vi "ManMarkZagueiro.vi"(8 "Our Robot":T1={"id"=0, "function"=enum."Attacker", "x"=0.0, "y"=0.0, "orientation"=0.0, "v_tangent"=0.0, "v_normal"=0.0, "v_ang"=0.0, "kick_x"=0.0, "kick_z"=0.0, "dribble"=FALSE, "Timestamp"=timestamp(0 s since 1904-01-01), "estimatives"={"est_v_tangent"=0.0, "est_v_normal"=0.0, "est_vx"=0.0, "est_vy"=0.0, "Pos Robot Est"=[]}, "dest_x_kick"=0.0, "dest_y_kick"=0.0, "Gap Coord"=[], "States"=enum."GoToTangent", "Path "=[], "Path  Smooth"=[], "Dest"=[]}, 10 "IA Input":T6={"our_robots"=[], "enemy_robots"=[], "balls"=[], "geometry"={"line_width"=0, "field_length"=0, "field_width"=0, "boundary_width"=0, "referee_width"=0, "goal_width"=0, "goal_depth"=0, "goal_wall_width"=0, "center_circle_radius"=0, "defense_radius"=0, "defense_stretch"=0, "free_kick_from_defense_dist"=0, "penalty_spot_from_field_line_dist"=0, "penalty_line_from_spot_dist"=0}, "IA Judge"={"stage"="", "command"="", "our_goalie_id"=0.0, "enemy_goalie_id"=0.0, "command enum"=enum."Halt", "Time"=enum."Azul"}, "Received Timestamp"=timestamp(0 s since 1904-01-01), "Events"={"Touch"=FALSE, "Ball out"=FALSE, "id touch"=0.0, "Ball out of \nVision"=FALSE, "Ball inside \nGoalie area"=FALSE, "Robot not responding"=FALSE, "Robots responding status"=[1.0, 1.0, 1.0, 1.0, 1.0, 1.0], "Enemy Ball \nPossession"=FALSE, "Pass State"=FALSE, "id end of pass"=0.0, "Kick"=FALSE, "Id ini Possession"=0.0, "Ball Possesion"=FALSE, "Id Possesion"=0.0}}) -> (2 "Robot out":T1={"id"=0, "function"=enum."Attacker", "x"=0.0, "y"=0.0, "orientation"=0.0, "v_tangent"=0.0, "v_normal"=0.0, "v_ang"=0.0, "kick_x"=0.0, "kick_z"=0.0, "dribble"=FALSE, "Timestamp"=timestamp(0 s since 1904-01-01), "estimatives"={"est_v_tangent"=0.0, "est_v_normal"=0.0, "est_vx"=0.0, "est_vy"=0.0, "Pos Robot Est"=[]}, "dest_x_kick"=0.0, "dest_y_kick"=0.0, "Gap Coord"=[], "States"=enum."GoToTangent", "Path "=[], "Path  Smooth"=[], "Dest"=[]})   [LabVIEW 2017]
uses:
  Core/AI Input.ctl
  Core/AI Robot.ctl
  Functions Enum.ctl
  AttackerStates.ctl
  Path Planning/RRT/PathDests.ctl
  Path Planning/RRT/PathDest.ctl
  Core/AI Ball.ctl
  Core/Field Size.ctl
  Core/AI Judge.ctl
  Command Enum.ctl
  Util/Events/Events.ctl
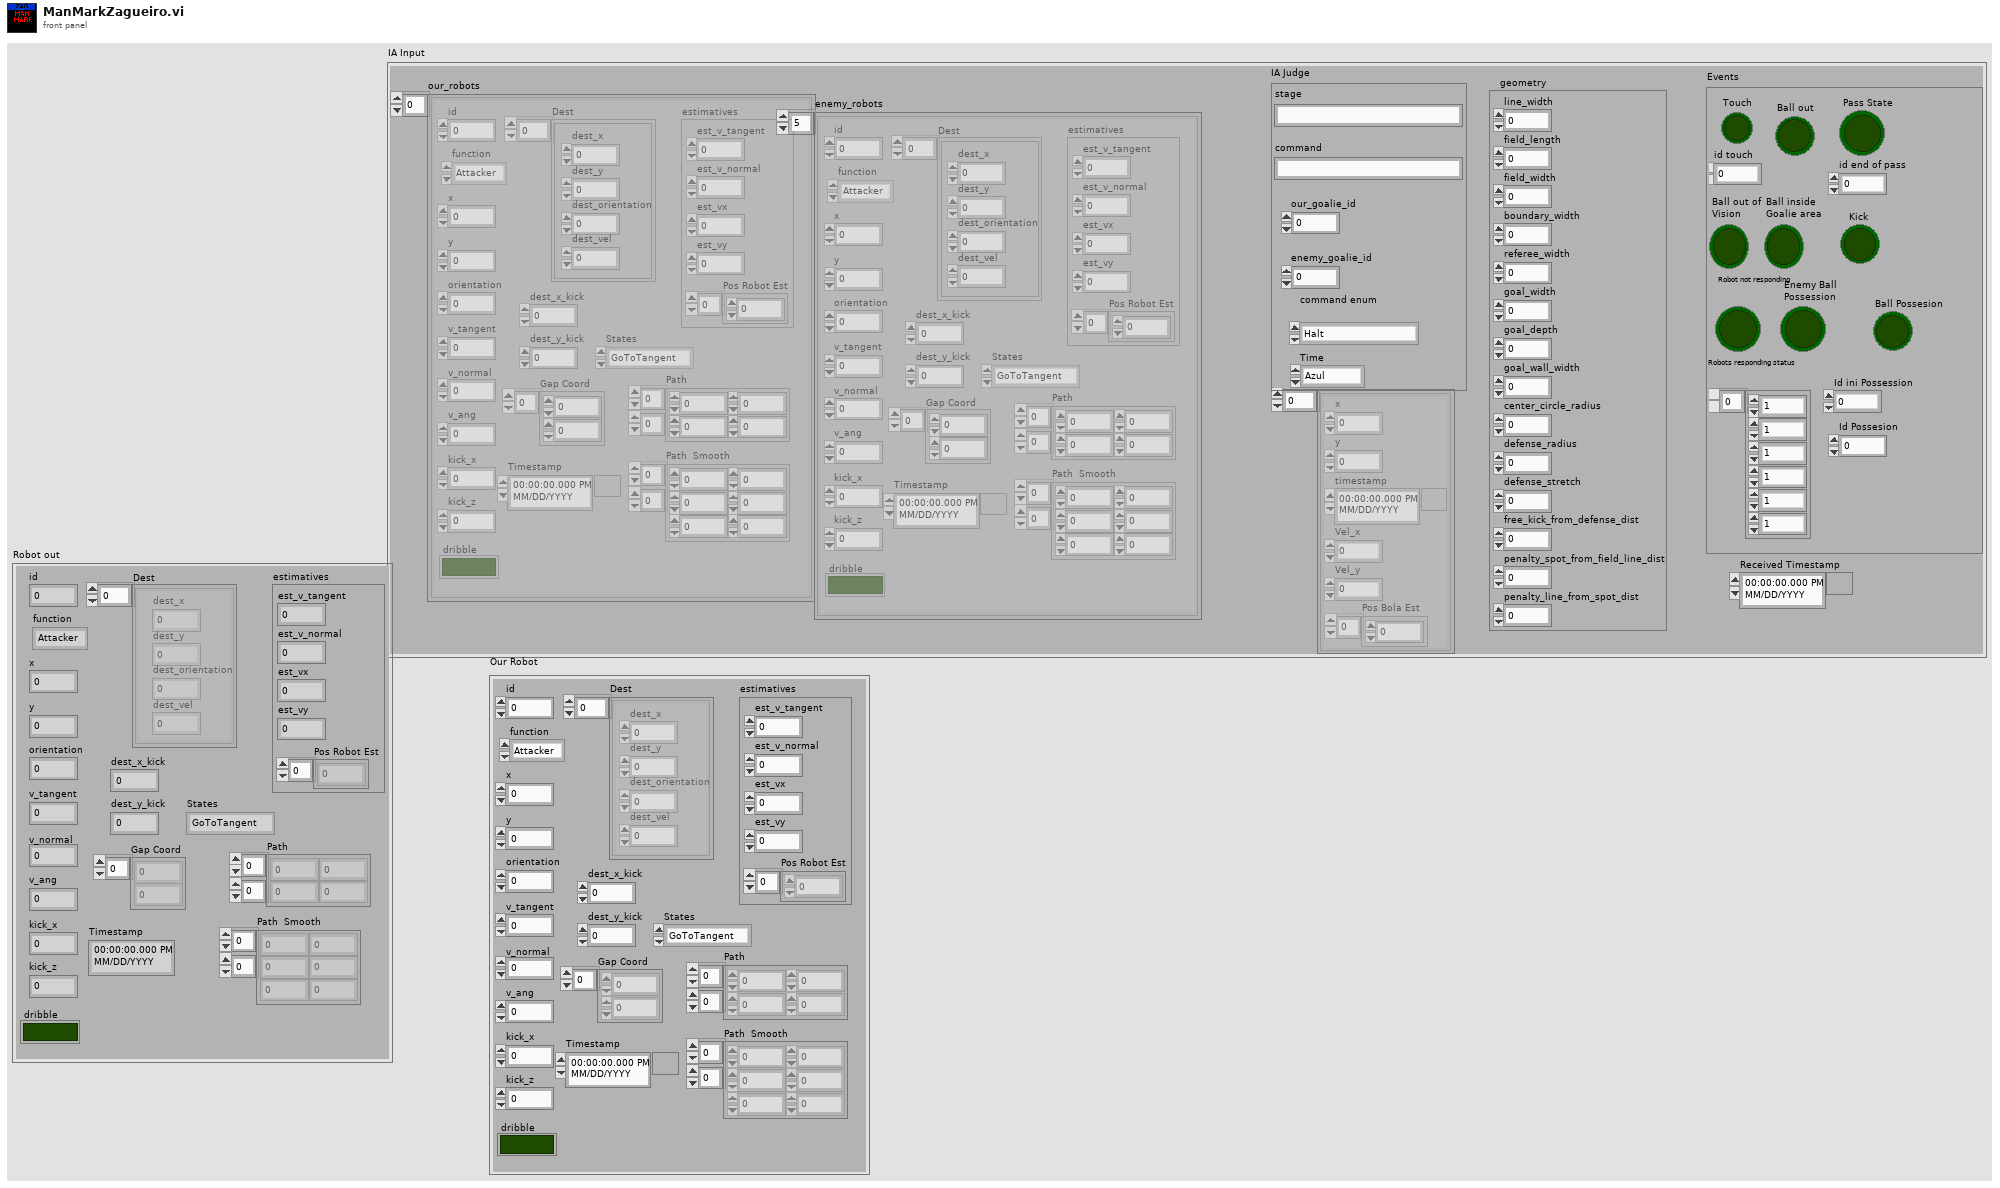
[diagram p1: front panel]
types:
  T1 = typedef "AI Robot.ctl" = cluster{"id":u32, "function":T2, "x":dbl, "y":dbl, "orientation":dbl, "v_tangent":dbl, "v_normal":dbl, "v_ang":dbl, "kick_x":dbl, "kick_z":dbl, "dribble":bool, "Timestamp":timestamp, "estimatives":cluster{"est_v_tangent":dbl, "est_v_normal":dbl, "est_vx":dbl, "est_vy":dbl, "Pos Robot Est":dbl[]}, "dest_x_kick":dbl, "dest_y_kick":dbl, "Gap Coord":dbl[], "States":T3, "Path ":dbl[][], "Path  Smooth":dbl[][], "Dest":T4}
  T2 = typedef "Functions Enum.ctl" = enum16{"Attacker", "Goalie", "Defender", "Striker", "Goto 0", "Dummy", "Kicker", "ZigZag"}
  T3 = typedef "AttackerStates.ctl" = enum16{"Pass", "GoToTangent", "BallGetting", "GoToKick", ""}
  T4 = typedef "PathDests.ctl" = T5[]
  T5 = typedef "PathDest.ctl" = cluster{"dest_x":dbl, "dest_y":dbl, "dest_orientation":dbl, "dest_vel":dbl}
  T6 = typedef "AI Input.ctl" = cluster{"our_robots":T1[], "enemy_robots":T1[], "balls":T7[], "geometry":T8, "IA Judge":T9, "Received Timestamp":timestamp, "Events":T11}
  T7 = typedef "AI Ball.ctl" = cluster{"x":dbl, "y":dbl, "timestamp":timestamp, "Vel_x":dbl, "Vel_y":dbl, "Pos Bola Est":dbl[]}
  T8 = typedef "Field Size.ctl" = cluster{"line_width":u32, "field_length":u32, "field_width":u32, "boundary_width":u32, "referee_width":u32, "goal_width":u32, "goal_depth":u32, "goal_wall_width":u32, "center_circle_radius":u32, "defense_radius":u32, "defense_stretch":u32, "free_kick_from_defense_dist":u32, "penalty_spot_from_field_line_dist":u32, "penalty_line_from_spot_dist":u32}
  T9 = typedef "AI Judge.ctl" = cluster{"stage":string, "command":string, "our_goalie_id":dbl, "enemy_goalie_id":dbl, "command enum":T10, "Time":enum16{"Azul", "Amarelo"}}
  T10 = typedef "Command Enum.ctl" = enum16{"Halt", "Stop", "Force Start", "PKA Normal Start", "Prepare Kickoff Ally", "PKE Normal Start", "Prepare Kickoff Enemy", "Prepare Penalty Ally", "PPA Normal Start", "Prepare Penalty Enemy", "PPE Normal Start", "Direct Free Enemy", "Direct Free Ally", "Indirect Free Enemy", "Indirect Free Ally", "Timeout Enemy", "Timeout Ally", "Goal Enemy", "Goal Ally", "Ball Placement Enemy", "Ball Placement Ally", "Normal Half Time", "Extra Time Break", "Extra Half Time", "None", "Post Game"}
  T11 = typedef "Events.ctl" = cluster{"Touch":bool, "Ball out":bool, "id touch":dbl, "Ball out of \nVision":bool, "Ball inside \nGoalie area":bool, "Robot not responding":bool, "Robots responding status":dbl[], "Enemy Ball \nPossession":bool, "Pass State":bool, "id end of pass":dbl, "Kick":bool, "Id ini Possession":dbl, "Ball Possesion":bool, "Id Possesion":dbl}
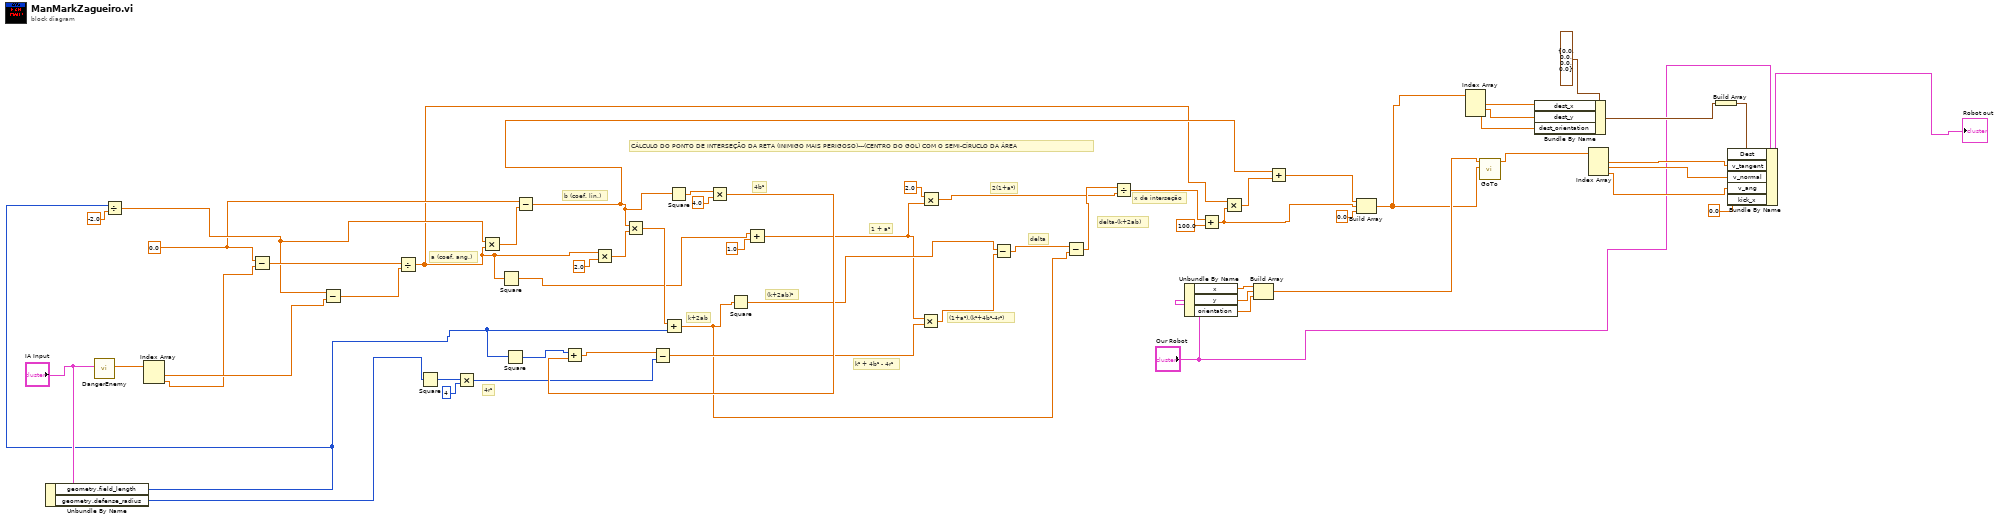
[diagram p0: block diagram]
diagram:
  w32 = 0.0
  # "x de interseção"
  # "CÁLCULO DO PONTO DE INTERSEÇÃO DA RETA (INIMIGO MAIS PERIGOSO)---(CENTRO DO GOL) COM O SEMI-CÍRUCLO DA ÁREA"
  # "delta-(k+2ab)"
  # "2(1+a²)"
  # "delta"
  # "(1+a²).(k²+4b²-4r²)"
  # "(k+2ab)²"
  # "k+2ab"
  # "k² + 4b² - 4r²"
  # "1 + a²"
  # "4r²"
  # "4b²"
  # "b (coef. lin.)"
  # "a (coef. ang.)"
  n1 = Unbundle By Name("IA Input") -> ("geometry.field_length"=w3:u32, "geometry.defense_radius"=w2:u32)
  n2 = call "DangerEnemy.vi"("IA Input"="IA Input") -> ("Pos do inimigo\nperigoso"=w31:dbl[])  [unwired: 7 in, 3 out]
  n3 = Divide(x=w3, y=-2.0) -> (x/y=w33:dbl)
  n4 = Index Array(array=w31) -> (element #1=w30:dbl, element #2=w29:dbl)  [unwired: 2 in]
  n5 = Subtract(x=w32, y=w29) -> (x-y=w60:dbl)
  n6 = Subtract(x=w33, y=w30) -> (x-y=w59:dbl)
  n7 = Divide(x=w60, y=w59) -> (x/y=w26:dbl)
  n8 = Square(x=w2) -> (x^2=w48:u32)
  n9 = Multiply(x=w48, y=u32 4) -> (x*y=w35:u32)
  n10 = Multiply(x=w33, y=w26) -> (x*y=w58:dbl)
  n11 = Square(x=w26) -> (x^2=w53:dbl)
  n12 = Square(x=w3) -> (x^2=w52:u32)
  n13 = Subtract(x=w32, y=w58) -> (x-y=w36:dbl)
  n14 = Multiply(x=w26, y=2.0 ("x")) -> (x*y=w56:dbl)
  n15 = Multiply(x=w36, y=w56) -> (x*y=w55:dbl)
  n16 = Add(x=w55, y=w3) -> (x+y=w41:dbl)
  n17 = Square(x=w36) -> (x^2=w51:dbl)
  n18 = Multiply(x=w51, y=4.0 ("x")) -> (x*y=w49:dbl)
  n19 = Add(x=w52, y=w49) -> (x+y=w46:dbl)
  n20 = Subtract(x=w46, y=w35) -> (x-y=w45:dbl)
  n21 = Square(x=w41) -> (x^2=w44:dbl)
  n22 = Add(x=w53, y=1.0) -> (x+y=w40:dbl)
  n23 = Multiply(x=w40, y=w45) -> (x*y=w43:dbl)
  n24 = Multiply(x=2.0 ("y"), y=w40) -> (x*y=w37:dbl)
  n25 = Subtract(x=w44, y=w43) -> (x-y=w42:dbl)
  n26 = Subtract(x=w42, y=w41) -> (x-y=w38:dbl)
  n27 = Divide(x=w38, y=w37) -> (x/y=w27:dbl)
  n28 = Unbundle By Name("Our Robot") -> ("x"=w21:dbl, "y"=w20:dbl, "orientation"=w19:dbl)
  n29 = Add(x=w27, y=100.0) -> (x+y=w23:dbl)
  n30 = Multiply(x=w26, y=w23) -> (x*y=w25:dbl)
  n31 = Build Array(w21, w20, w19) -> (w18:dbl[])
  n32 = Add(x=w36, y=w25) -> (x+y=w24:dbl)
  n33 = Build Array(w24, w23, 0.0 ("element")) -> (w16:dbl[])
  n34 = Index Array(array=w16) -> (element #1=w14:dbl, element #2=w13:dbl, element #3=w12:dbl)  [unwired: 3 in]
  n35 = call "GoTo.vi"("Target"=w16, "Position"=w18) -> ("Output\nVelocity"=w17:dbl[])  [unwired: 8 in, 1 out]
  n36 = Bundle By Name(cluster=T5 {"dest_x"=0.0, "dest_y"=0.0, "dest_orientation"=0.0, "dest_vel"=0.0} ("element"), "dest_x"=w14, "dest_y"=w13, "dest_orientation"=w12) -> (w10:T5)
  n37 = Index Array(array=w17) -> (element #1=w9:dbl, element #2=w8:dbl, element #3=w7:dbl)  [unwired: 3 in]
  n38 = Build Array(w10) -> (w11:T5[])
  n39 = Bundle By Name(cluster="Our Robot", "Dest"=w11, "v_tangent"=w9, "v_normal"=w8, "v_ang"=w7, "kick_x"=0.0) -> (→"Robot out":T1)
